vi "Generate Actions Tree.vi"(8 "error in (no error)":errorcluster, 11 "Tree Refnum IN":refnum<vi>) -> (0 "error out":errorcluster)   [LabVIEW 2012]
doc: "SciScan 1.2 160622"
uses:
  Custom Controls/MAIN Image panel tab Control type def.ctl
panel:
  in  "Tree":string(tree)
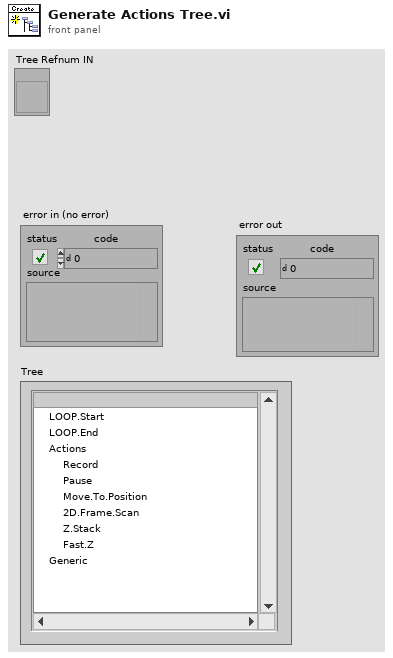
[diagram p1: front panel]
types:
  T1 = typedef "MAIN Image panel tab Control type def.ctl" = enum32{"Channel 1", "Channel 2", "Channel 3", "Channel 4", "all channels", "RGB overlay", "ROI", "arbitrary line scan"}
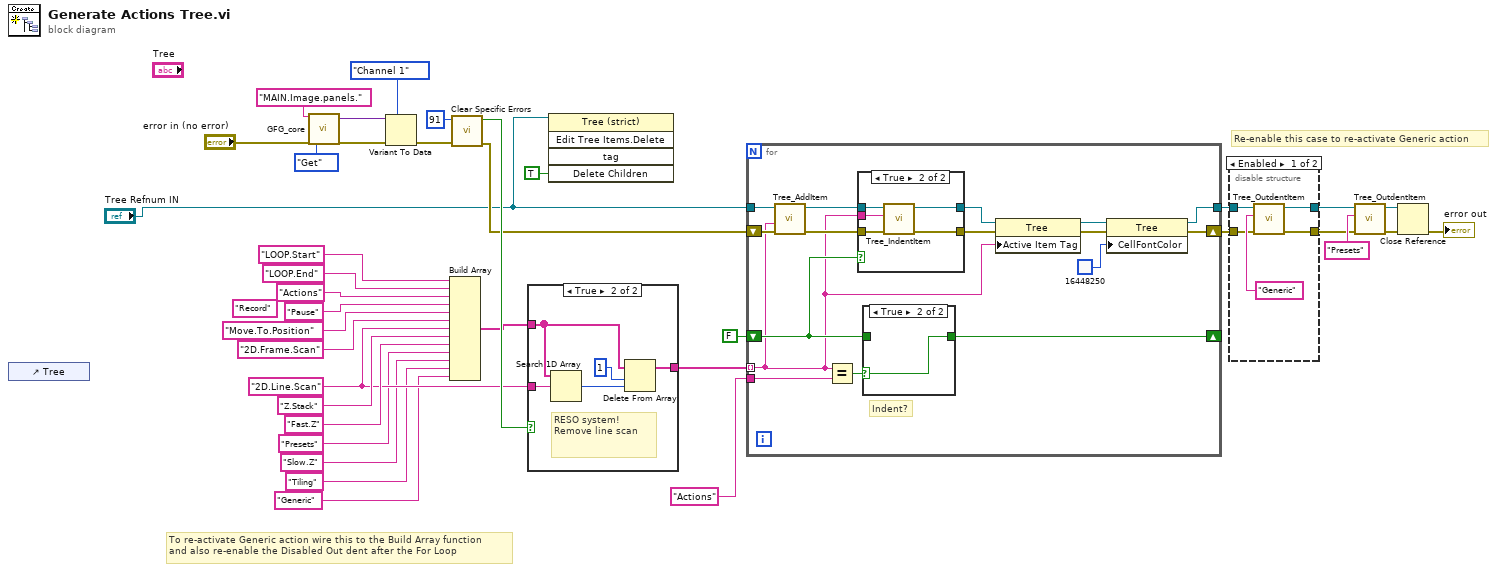
[diagram p0: block diagram]
diagram:
  w20 = "2D.Line.Scan"
  (unwired) "Record"
  # "To re-activate Generic action wire this to the Build Array function\nand also re-enable the Disabled Out dent after the For Loop"
  # "Re-enable this case to re-activate Generic action"
  n1 = control-ref of="Tree"() -> ()  [unwired: 1 out]
  n2 = call "GFG_core.vi"("Variable Name in"="MAIN.Image.panels.", "error in (no error)"="error in (no error)", "Action"=enum16{"Init", "Set", "Get", "Clear"}."Get") -> ("Variant Out"=w27:variant, "error out"=w24:errorcluster)  [unwired: 10 in, 5 out]
  n3 = Variant To Data(error in=w24, type=MAIN_Image_panel_tab_Control_type_def."Channel 1" ("MAIN Image panels"), Variant=w27) -> (error out=w28:errorcluster)  [unwired: 1 out]
  n4 = Build Array("LOOP.Start", "LOOP.End", "Actions", "Pause", "Move.To.Position", "2D.Frame.Scan", w20, "Z.Stack", "Fast.Z", "Presets", "Slow.Z", "Tiling", "Generic") -> (w21:string[])
  n5 = call "Clear Specific Errors.vi"("Error In"=w28, "Error number In"=91) -> ("Error Out"=w15:errorcluster, "Error Cleared?"=w22:bool)  [unwired: 8 in]
  n6 = case shown="True" w22 {
    tunnel: w21 -> [w38 w42]
    tunnel: w20 -> [_ w43]
    tunnel: [w38 w39] -> w19
    frame False {
    }
    frame True {
      # "RESO system!\nRemove line scan"
      n7 = Search 1D Array(1D array=w42, element=w43) -> (index of element=w40:i32)  [unwired: 1 in]
      n8 = Delete From Array(array=w42, length=1, index=w40) -> (array with subset deleted=w39:string[])  [unwired: 1 out]
    }
  }
  n9 = invoke class="Tree (strict)" method="Edit Tree Items.Delete"(reference="Tree Refnum IN", "Delete Children"=TRUE ("Delete Children?")) -> ()  [unwired: 3 in, 5 out]
  n10 = for {
    tunnel: "Tree Refnum IN" -> [w59]
    tunnel: w19 -> [w48] mode=indexing
    tunnel: "Actions" -> [w58]
    shift-right: [w55] -> _
    shift-left: FALSE -> [w54]
    tunnel: [w44] -> w16
    shift-right: [w45] -> w14
    shift-left: w15 -> [w52]
    # "Indent?"
    n11 = call "Tree_AddItem.vi"("Error In"=w52, "NEW String"=w48, "Tree Refnum"=w59) -> ("Error Out"=w53:errorcluster, "Tree Refnum OUT"=w57:refnum<vi>)  [unwired: 6 in, 1 out]
    n12 = Equal?(x=w48, y=w58) -> (x = y?=w56:bool)
    n13 = case shown="True" w54 {
      tunnel: w57 -> [w63 w68]
      tunnel: w48 -> [_ w67]
      tunnel: [w63 w66] -> w50
      tunnel: w53 -> [w62 w65]
      tunnel: [w62 w64] -> w49
      frame False {
      }
      frame True {
        n14 = call "Tree_IndentItem.vi"("Error In"=w65, "TagToIndent"=w67, "Tree Refnum"=w68) -> ("Error Out"=w64:errorcluster, "Tree Refnum OUT"=w66:refnum<vi>)  [unwired: 7 in]
      }
    }
    n15 = case shown="True" w56 {
      selector: w56 -> [_ w61]
      tunnel: [w60 w61] -> w55
      tunnel: w54 -> [w60 _]
      frame False {
      }
      frame True {
      }
    }
    n16 = property class="Tree"(reference=w50, error in=w49, "Active Item Tag"=w48) -> (reference out=w46:refnum<vi>, error out=w47:errorcluster)
    n17 = property class="Tree"(reference=w46, error in=w47, "CellFontColor"=u32 16448250) -> (reference out=w44:refnum<vi>, error out=w45:errorcluster)
  }
  n18 = disable-structure shown="Enabled" {
    disable-tunnel: w16 -> [w73 w75]
    disable-tunnel: w14 -> [w71 w74]
    disable-tunnel: [w70 w74] -> w6
    disable-tunnel: [w69 w75] -> w5
    frame Enabled {
      n19 = call "Tree_OutdentItem.vi"("Error In"=w71, "TagToOutdent"="Generic", "Tree Refnum"=w73) -> ("Error Out"=w70:errorcluster, "Tree Refnum OUT"=w69:refnum<vi>)  [unwired: 7 in]
    }
    frame Disabled {
    }
  }
  n20 = call "Tree_OutdentItem.vi"("Error In"=w6, "TagToOutdent"="Presets", "Tree Refnum"=w5) -> ("Error Out"=w3:errorcluster, "Tree Refnum OUT"=w4:refnum<vi>)  [unwired: 7 in]
  n21 = Close Reference(reference=w4, error in (no error)=w3) -> (error out=→"error out":errorcluster)
